vi "Localization-StaticDemo.vi"() -> ()   [LabVIEW 2010]
doc: "本地化演示"
panel:
  out "String":string caption="字符串"
  in  "Ring":u16(ring) caption="下拉列表框" items=["加载", "卸载", "打开", "关闭"]
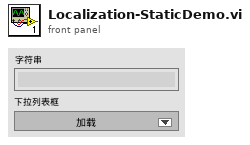
[diagram p1: front panel]
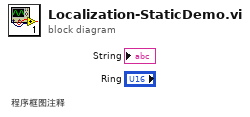
[diagram p0: block diagram]
diagram:
  # "程序框图注释"
